vi "Get Key Value (Variant).vi"(5 "Key name":string, 6 "Default value":variant, 7 "Section name":string, 8 "error in (no error)":errorcluster, 9 "Use LV Default? [F]":bool, 10 "Strip Whitespace? [T]":bool=TRUE, 11 "Carya Config in":refnum<class "Carya Config.lvclass">) -> (0 "error out":errorcluster, 1 "Found?":bool, 2 "Value":variant, 3 "Carya Config out":refnum<class "Carya Config.lvclass">)   [LabVIEW 2013, in "Carya Config.lvclass"]
doc: "Copyright 2018, Carya Automatisering, Wiebe Walstra."
uses:
  Carya Config.lvclass
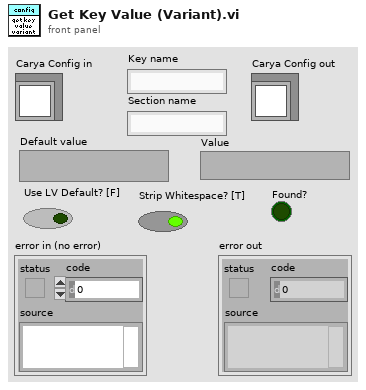
[diagram p1: front panel]
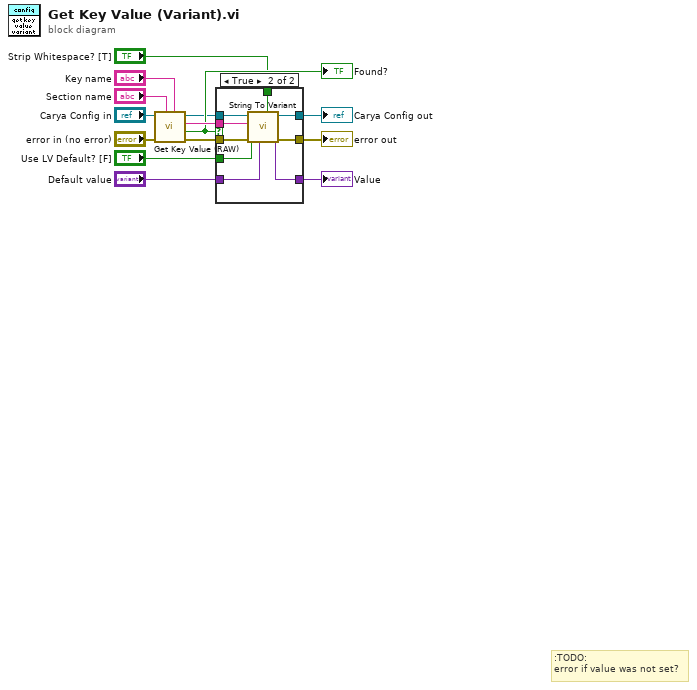
[diagram p0: block diagram]
diagram:
  # ":TODO:\nerror if value was not set?"
  n1 = call-dynamic "Get Key Value (RAW).vi"("Key name"="Key name", "Section name"="Section name", "error in (no error)"="error in (no error)", "Carya Config in"="Carya Config in") -> ("error out"=w13:errorcluster, "Found?"=w6:bool, "Value"=w8:string, "Carya Config out"=w4:refnum<class "Carya Config.lvclass">)  [unwired: 4 in]
  "Found?" <- w6
  n2 = case shown="True" w6 {
    tunnel: w13 -> [w16 w23]
    tunnel: [w16 w26] -> w9
    tunnel: w8 -> [_ w24]
    tunnel: "Default value" -> [w17 w22]
    tunnel: [w17 w25] -> w5
    tunnel: w4 -> [w15 w21]
    tunnel: [w15 w20] -> w3
    tunnel: "Use LV Default? [F]" -> [_ w19]
    tunnel: "Strip Whitespace? [T]" -> [_ w18]
    frame False {
    }
    frame True {
      n3 = call-dynamic "String To Variant.vi"("Strip Whitespace? [T]"=w18, "Variant Type\\default"=w22, "error in (no error)"=w23, "Use LV Default? [F]"=w19, "String"=w24, "Registry Object"=w21) -> ("error out"=w26:errorcluster, "Variant"=w25:variant, "Registry Object"=w20:refnum<class "Carya Config.lvclass">)  [unwired: 3 in]
    }
  }
  "error out" <- w9
  "Carya Config out" <- w3
  "Value" <- w5
